vi "Init.vi"() -> ()   [LabVIEW 2020]
uses:
  <vilib>/Utility/sysdir.llb/System Directory Type.ctl
panel:
  in  "error in (no error)":errorcluster
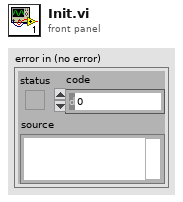
[diagram p1: front panel]
types:
  T1 = typedef "System Directory Type.ctl" = i32
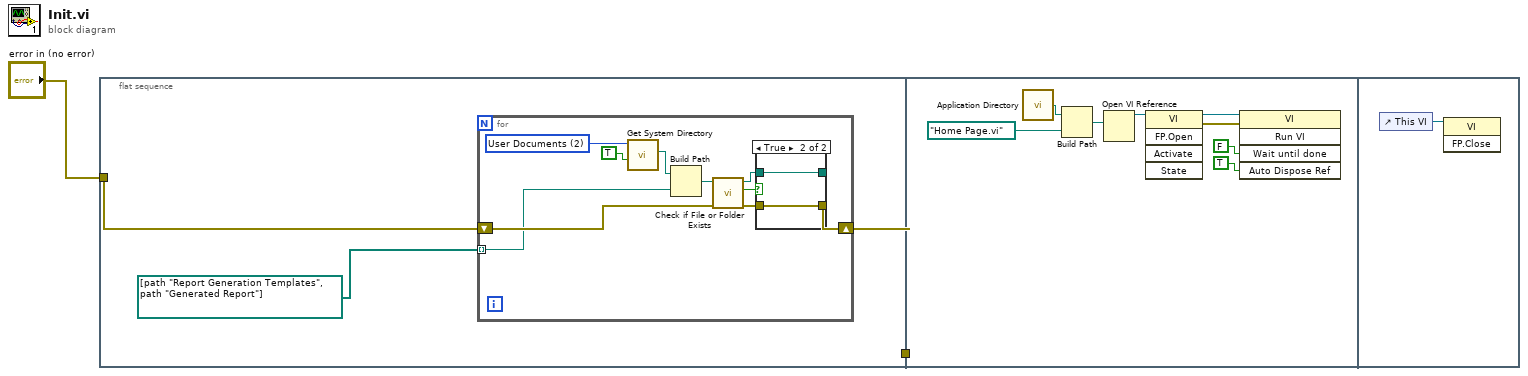
[diagram p0: block diagram]
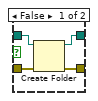
[diagram p2: hidden frame]
diagram:
  n1 = flat-sequence {
    tunnel: "error in (no error)" -> [w5]
    tunnel: [w4] -> w1
    tunnel: w1 -> [_]
    frame #0 {
      n2 = for {
        tunnel: path[] [path "Report Generation Templates", path "Generated Report"] -> [w7] mode=indexing
        shift-right: [w9] -> w4
        shift-left: w5 -> [w13]
        w15 = T1 2 items=["User Home"=0, "User Desktop"=1, "User Documents"=2, "User Application Data"=3, "User Preferences"=4, "User Temporary"=5, "Public Documents"=6, "Public Application Data"=7, "Public Preferences"=8, "Public Cache"=13, "System Core Libraries"=9, "System Installed Libraries"=10, "Application Files"=11, "Boot Volume Root"=12] ("system directory type")
        n3 = call <vilib>:"Get System Directory.vi"("create directory if not found? (F)"=TRUE, "system directory type"=w15) -> ("system directory"=w8:path)  [unwired: 9 in]
        n4 = Build Path(base path=w8, name or relative path=w7) -> (appended path=w6:path)
        n5 = call <vilib>:"Check if File or Folder Exists.vi"("error in (no error)"=w13, "path"=w6) -> ("error out"=w10:errorcluster, "file or folder exists?"=w11:bool, "dup path"=w12:path)  [unwired: 7 in]
        n6 = case shown="True" w11 {
          tunnel: w12 -> [w19 w21]
          tunnel: w10 -> [w18 w20]
          tunnel: [w17 w20] -> w9
          tunnel: [w16 w21] -> _
          frame False {
            n7 = Create Folder(path (use dialog)=w19, error in=w18) -> (created path=w16:path, error out=w17:errorcluster)  [unwired: 1 in, 1 out]
          }
          frame True {
          }
        }
      }
    }
    frame #1 {
      n8 = call <vilib>:"Application Directory.vi"() -> ("Application Directory"=w29:path)
      n9 = Build Path(base path=w29, name or relative path=path "Home Page.vi") -> (appended path=w27:path)
      n10 = Open VI Reference(vi path=w27) -> (vi reference=w26:refnum<vi>)  [unwired: 5 in, 1 out]
      n11 = invoke class="VI" method="FP.Open"(reference=w26) -> (reference out=w25:refnum<vi>, error out=w24:errorcluster)  [unwired: 4 in, 3 out]
      n12 = invoke class="VI" method="Run VI"(reference=w25, error in=w24, "Wait until done"=FALSE ("Wait Until Done"), "Auto Dispose Ref"=TRUE ("Auto Dispose Reference")) -> ()  [unwired: 1 in, 5 out]
    }
    frame #2 {
      n13 = control-ref of="This VI"() -> (w30:refnum<vi>)
      n14 = invoke class="VI" method="FP.Close"(reference=w30) -> ()  [unwired: 2 in, 3 out]
    }
  }
